vi "Average Shooter Distance.vi"(11 "Distance Values (in)":dbl[](array[numeric])) -> (1 "Distance Values (out)":dbl[](array[numeric]), 2 "Average Distance":dbl, 3 "Distance (ft)":dbl)   [LabVIEW 2016]
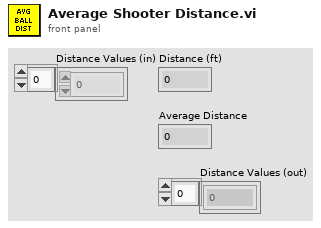
[diagram p1: front panel]
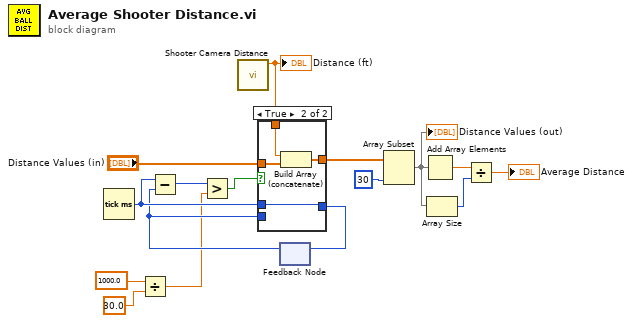
[diagram p0: block diagram]
diagram:
  n1 = Tick Count (ms)() -> (millisecond timer value=w7:u32)
  n2 = Divide(x=1000.0, y=30.0) -> (x/y=w1:dbl)
  n3 = call "Shooter Camera Distance.vi"() -> ("Distance (ft)"=w16:dbl)  [unwired: 9 in, 2 out]
  "Distance (ft)" <- w16
  n4 = feedback #1() -> (w6:u32)  [unwired: 1 in]
  n5 = Subtract(x=w7, y=w6) -> (x-y=w5:u32)
  n6 = Greater?(x=w5, y=w1) -> (0:w4:bool)
  n7 = case shown="True" w4 {
    tunnel: w16 -> [_ w22]
    tunnel: "Distance Values (in)" -> [w18 w21]
    tunnel: [w18 w20] -> w9
    tunnel: w7 -> [_ w19]
    tunnel: [w17 w19] -> w8
    tunnel: w6 -> [w17 _]
    frame False {
    }
    frame True {
      n8 = Build Array (concatenate)(w22, w21) -> (w20:dbl[])
    }
  }
  n9 = feedback-in #1(w8) -> ()
  n10 = Array Subset(array=w9, length=30) -> (w13:dbl[])  [unwired: 1 in]
  "Distance Values (out)" <- w13
  n11 = Add Array Elements(numeric array=w13) -> (sum=w10:dbl)
  n12 = Array Size(array=w13) -> (size(s)=w11:i32)
  n13 = Divide(x=w10, y=w11) -> (x/y=→"Average Distance":dbl)
